vi "LVClass_ModalCoef SetZernikePrefs.vi"(0 "ModalCoef in":refnum<class "ModalCoef.lvclass">, 5 "ZernikeModalPrefs":T1={"Number of coefficients"=32, "Filtered coefficients"=[], "RMS Zernike normalization"=FALSE, "CircularProjectionPupilDimensions"={"Pupil center_sspp"={"X"=0.0, "Y"=0.0}, "Pupil radius_sspp"=0.0}}, 11 "error in (no error)":errorcluster) -> (4 "ModalCoef out":refnum<class "ModalCoef.lvclass">, 15 "error out":errorcluster)   [LabVIEW 2020, in "ModalCoef.lvclass"]
doc: "Set the Zernike preferences for modal phase reconstruction.\n\n--------------------------------------------------------------------------------\n\n<B>ComputePhaseSetIn </B> : ComputePhaseSet object.\n<B>ComputePhaseSetOut </B> : ComputePhaseSet object.\n<B>normalisation </B> : Normalisation Phase coefficients enumeration :\n * 0 : standard\n * 1 : rms\n<B>nb_coeffs_total </B> : Number of the Zernike coefficients used in the polynomial base.\n<B>nb_coeffs_to_filter </B> : Number of the Zernike coefficients to filter in the polynomial base.\n<B>coeffs_to_filter </B> : List of indices of the Zernike coefficients to filter in the polynomial base.\n<B>projection_pupil_center </B> : Center of the projection pupil, in number of subpupils.\n<B>projection_pupil_radius </B> : Projection pupil radius, in number of subpupils.\n<B>ErrorIn </B> : Error\n<B>ErrorOut </B> : Error\n\n--------------------------------------------------------------------------------"
uses:
  ModalCoef.lvclass
  Controls/ZernikeModalPrefs.ctl
  Controls/ZernikeProjectionPupilSetup.ctl
  Controls/Point2Df.ctl
  ModalCoef.lvclass/ModalCoef.ctl
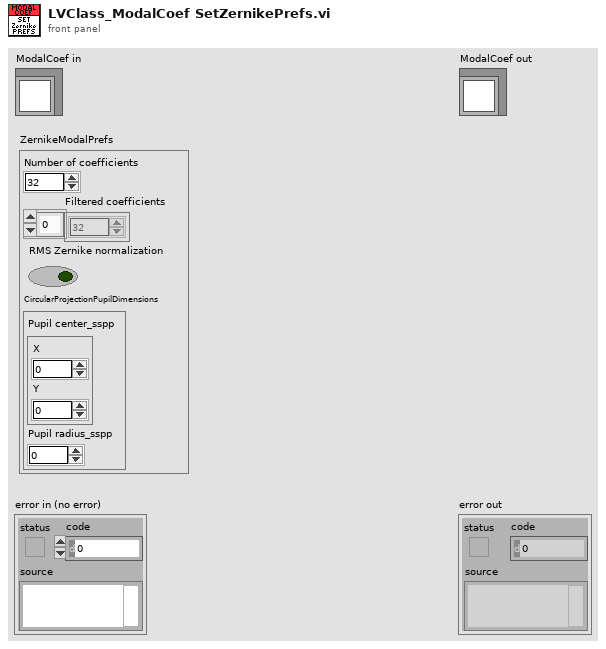
[diagram p1: front panel]
types:
  T1 = typedef "ZernikeModalPrefs.ctl" = cluster{"Number of coefficients":u32, "Filtered coefficients":u32[], "RMS Zernike normalization":bool, "CircularProjectionPupilDimensions":T2}
  T2 = typedef "ZernikeProjectionPupilSetup.ctl" = cluster{"Pupil center_sspp":T3, "Pupil radius_sspp":sgl}
  T3 = typedef "Point2Df.ctl" = cluster{"X":sgl, "Y":sgl}
  T4 = typedef "ClassID.ctl" = i64
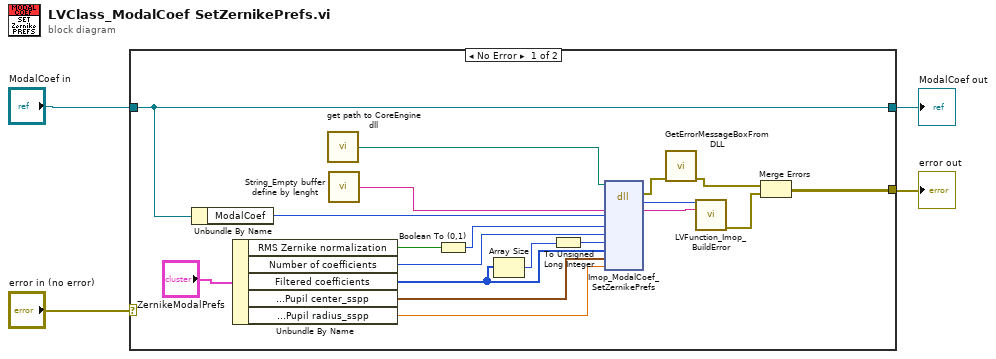
[diagram p0: block diagram]
diagram:
  n1 = case shown="No Error" "error in (no error)" {
    selector: "error in (no error)" -> [_ w25]
    tunnel: [w5 w25] -> w1
    tunnel: [w9 w24] -> w3
    tunnel: "ModalCoef in" -> [w9 w24]
    frame No Error {
      n2 = Unbundle By Name(w9) -> ("ModalCoef"=w8:T4)
      n3 = Unbundle By Name("ZernikeModalPrefs") -> ("RMS Zernike normalization"=w17:bool, "Number of coefficients"=w15:u32, "Filtered coefficients"=w12:u32[], "CircularProjectionPupilDimensions.Pupil center_sspp"=w14:T3, "CircularProjectionPupilDimensions.Pupil radius_sspp"=w13:sgl)
      n4 = call "get path to CoreEngine dll.vi"() -> ("path to wavekit library"=w20:path)  [unwired: 14 in, 1 out]
      n5 = call "String_Empty buffer define by lenght.vi"() -> ("Empty buffer"=w21:string)  [unwired: 1 in]
      n6 = Boolean To (0,1)(Boolean=w17) -> (0, 1=w16:i16)
      n7 = Array Size(array=w12) -> (size(s)=w11:i32)
      n8 = To Unsigned Long Integer(number=w11) -> (unsigned 32bit integer=w10:u32)
      n9 = dll-call lib="D:/2_trunk/Soft_haso/ImOpCoreEngine4_LV2011/DLLs/ImopEngine4_vc100.dll" fn="Imop_ModalCoef_SetZernikePrefs"(path in=w20, "message"=w21, "objet"=w8, "normalisation"=w16, "numberOfCoefficient"=w15, "nb_polynomial_base_to_filter"=w10, "polynomial_base"=w12, "projection_pupil_center"=w14, "projection_pupil_diameter"=w13) -> (error out=w19:errorcluster, "return type"=w23:i32, "message"=w22:string)  [unwired: 9 in, 1 out]
      n10 = call "GetErrorMessageBoxFromDLL.vi"("error IN"=w19) -> ("error OUT"=w7:errorcluster)  [unwired: 10 in]
      n11 = call "LVFunction_Imop_BuildError.vi"("code"=w23, "String to Prepend to source (\"\")"=w22) -> ("error out"=w6:errorcluster)  [unwired: 13 in]
      n12 = Merge Errors(w7, w6) -> (w5:errorcluster)
    }
    frame Error {
    }
  }
  "error out" <- w1
  "ModalCoef out" <- w3
